vi "Controls - By List.vi"(7 "Msg Chain":string, 8 "error in (no error)":errorcluster {"code" format="Error %.0f"}, 10 "Controls Docs":refnum<class "GUI Documentation.lvclass">[](array[class]), 11 "VIDoc Printer - Confluence In":refnum<class "VIDoc Printer - Confluence.lvclass">) -> (0 "error out":errorcluster {"code" format="Error %.0f"}, 3 "VIDoc Printer - Confluence Out":refnum<class "VIDoc Printer - Confluence.lvclass">)   [LabVIEW 2023, in "VIDoc Printer - Confluence.lvlib" / "VIDoc Printer - Confluence.lvclass"]
uses:
  VIDoc Printer - Confluence.lvclass
  C:/projects/DMC/GitHub/DMC CLI VIDoc/Source/Documentation Generation/Printers/Printer/VIDoc Printer.lvclass
  Parsing/GUI Documentation/GUI Documentation.lvclass
  Confluence Formatting/Types/Format Combo Box.ctl
  Printer/VIDoc Printer.lvclass/VIDoc Printer.ctl
  VIDoc Printer - Confluence.lvclass/VIDoc Printer - Confluence.ctl
  Parsing/GUI Documentation/GUI Documentation.lvclass/GUI Documentation.ctl
  Types/VI Method Types.ctl
  Parsing/GUI Documentation/Get VI Info.vi
  Printer/Accessors/Get Formatting Settings - Bookmark Options.vi
  Printer/Accessors/Get Controls Settings - List Detail Level.vi
  Accessors/Get Sortable Tables.vi
  Accessors/Get Temporary Image Directory+.vi
  Accessors/Get Ctrls By List Expand.vi
  <vilib>/Utility/libraryn.llb/Create Directory Recursive.vi
  Confluence Formatting/Confluence Formatting.lvlib
  Printer/VIDoc Printer.lvclass
  UI Interaction/UI Interaction.lvclass
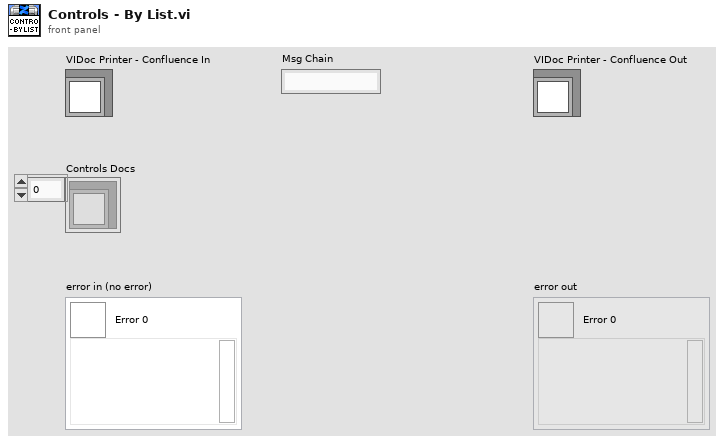
[diagram p1: front panel]
types:
  T1 = typedef "Confluence Formatting.lvlib/Format Combo Box.ctl" = string
  T2 = typedef "VIDoc Printer.lvlib/Printer Settings.lvclass/Bookmark Options.ctl" = cluster{"Bookmarks as New Line in VI Descriptions":bool, "Unique Bookmark Tags Only":bool, "Include Tag and Text":bool}
  T3 = typedef "VIDoc Printer.lvlib/Printer Settings.lvclass/Detail Level Enum.ctl" = enum16{"None", "Minimal", "Standard", "Full"}
  T4 = typedef "VIDoc Printer - Confluence.lvlib/VIDoc Printer - Confluence.lvclass/VI Method Types.ctl" = enum16{"Library", "Class", "Interface", "LLB", "UI", "List"}
  T5 = typedef "VIDoc Parsing.lvlib/Method Spec Cluster.ctl" = cluster{"VI Type Ext":T6, "Name":string, "Path":path, "Get Conpane Image":T7, "Description":string, "Get Library Access Scope":enum32{"invalid scope", "public", "private", "protected", "community"}, "Dispatch":T8, "ContainsCompiledCode":bool, "Exec.IsReentrant":bool, "Exec.ReentrancyType":enum16{"Share clones between instances", "Preallocate clone for each instance"}, "ExecInlining":bool, "ExecInlineIfPossible":bool, "Auto Err Handling":bool, "CodeComplexity":sgl, "Bookmark Tags":string[], "Control VI Type":enum32{"not a control VI", "control", "typedef", "strict typedef"}, "Controls":T9[], "VI Type":enum32{"invalid VI type", "Standard VI", "Control VI", "Global VI", "Polymorphic VI", "Configuration VI", "SubSystem", "Facade VI", "Method VI", "Statechart Diagram VI"}, "Minimum Size":T11, "Front Panel Window:Title":string, "Front Panel Window:Behavior":enum32{"Invalid", "Default", "Floating", "Floating/Auto-Hide", "Modal"}, "Front Panel Window:Closeable":bool, "Must Override":bool, "Must Use Parent Implementation":bool, "VI Icon":T7, "Front Panel":T7, "History:Revision Number":u32, "Metrics:Total Data Size":u32, "Execution:Allow Debugging":bool, "Execution:Preferred Exec System":enum32{"invalid execution system", "user interface", "standard", "instrument i/o", "data acquisition", "other 1", "other 2", "same as caller"}, "Execution:Priority":enum32{"invalid priority", "background priority", "normal priority", "above normal priority", "high priority", "time critical priority", "subroutine"}, "BM Tag Text":string[], "Block Diagram":T7, "Structure Tree":T12[]}
  T6 = typedef "VIDoc Parsing.lvlib/VI Type Extended Enum.ctl" = enum16{"Unknown", "Class Method", "Class Accessor Get", "Class Accessor Set", "Class Control", "Library Method", "Library Control", "VI", "Control"}
  T7 = typedef "imagedata.ctl" = cluster{"image type":i32, "image depth":i32, "image":u8[], "mask":u8[], "colors":u32[], "Rectangle":cluster{"left":i16, "top":i16, "right":i16, "bottom":i16}}
  T8 = typedef "VIDoc Parsing.lvlib/Class Dispatch Type Enum.ctl" = enum16{"None", "Static", "Dynamic"}
  T9 = typedef "VIDoc Parsing.lvlib/Controls Info Cluster.ctl" = cluster{"Name":string, "Description":string, "Data Type":string, "Tip Strip":string, "UID":i32, "Image Data":T7, "ToggleKeyBind":T10, "Raw Label":string, "Raw Caption":string}
  T10 = typedef "LVKeyTypeDef.ctl" = cluster{"Focus":bool, "Control":bool, "Shift":bool, "Key":string}
  T11 = typedef "LVPointTypeDef.ctl" = cluster{"Horizontal":i16, "Vertical":i16}
  T12 = typedef "VIDoc Parsing.lvlib/Structure Reporter.lvlib/Tree Cluster.ctl" = cluster{"Object Class Name":string, "Labels":string[], "Child Tag":string, "Item Indent":i32, "Child Only?":bool, "Glyph Index":i32}
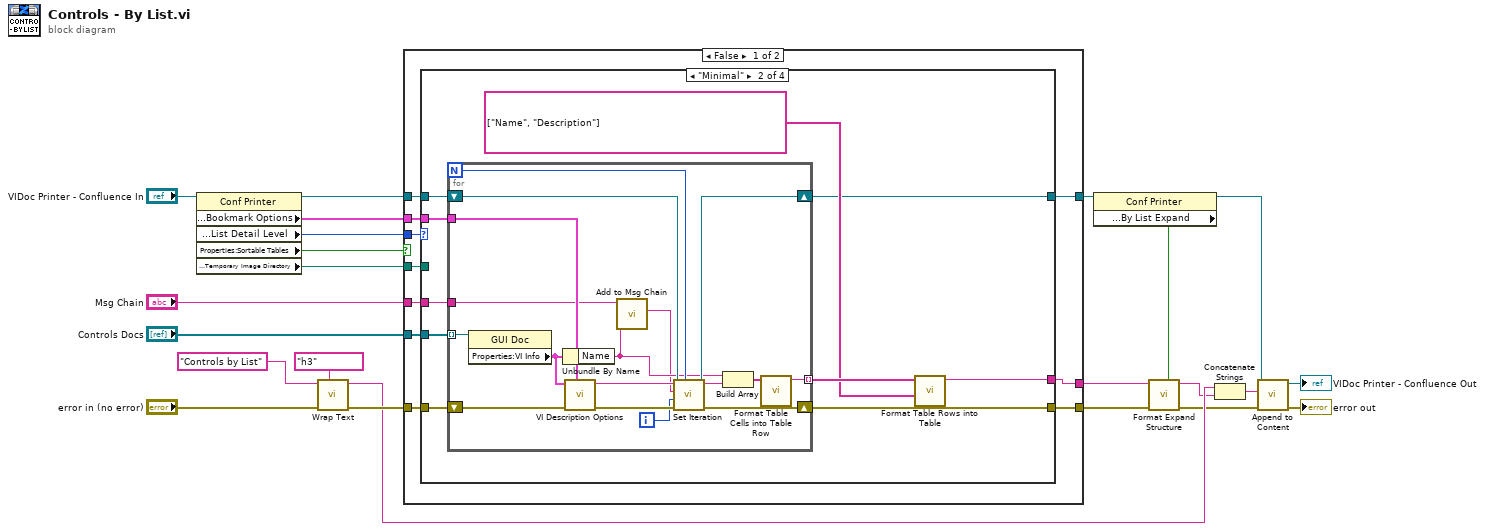
[diagram p0: block diagram]
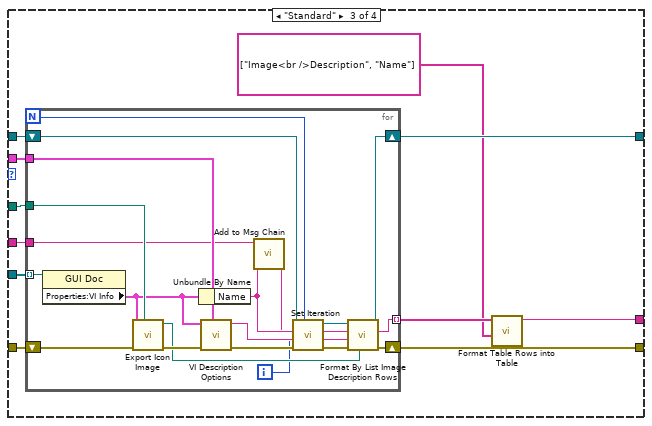
[diagram p3: hidden frame]
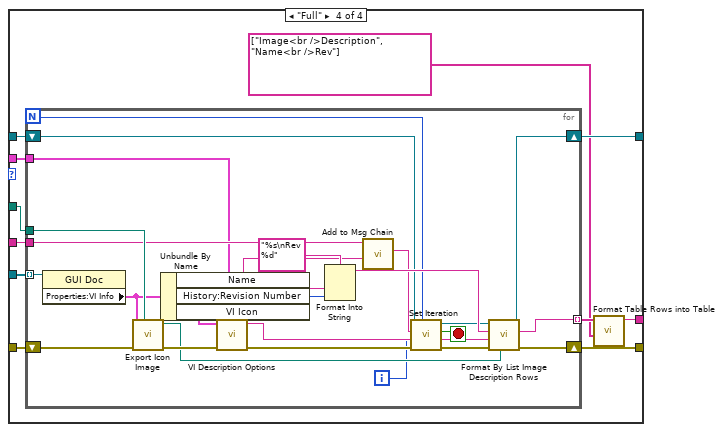
[diagram p4: hidden frame]
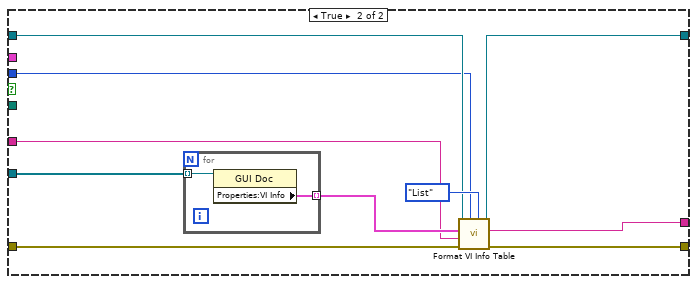
[diagram p5: hidden frame]
diagram:
  n1 = property class="Conf Printer"(reference="VIDoc Printer - Confluence In") -> (reference out=w20:refnum<class "VIDoc Printer - Confluence.lvclass">, "Properties:Settings:Formatting Options:Bookmark Options"=w9:T2, "Properties:Settings:Control Members:List Detail Level"=w8:T3, "Properties:Sortable Tables"=w2:bool, "Properties:Temporary Image Directory"=w1:path)  [unwired: 1 in, 1 out]
  n2 = call "Wrap Text.vi"("Formatting"=T1 "h3", "Error in"="error in (no error)", "String"="Controls by List" ("format string")) -> ("Error out"=w22:errorcluster, "Wrapped String"=w17:string)  [unwired: 7 in]
  n3 = case shown="False" w2 {
    tunnel: w22 -> [w33 w135]
    tunnel: [w32 w134] -> w21
    tunnel: w20 -> [w31 w132]
    tunnel: [w30 w128] -> w19
    tunnel: w1 -> [w29 _]
    tunnel: "Controls Docs" -> [w28 w129]
    tunnel: "Msg Chain" -> [w27 w130]
    tunnel: w9 -> [w26 _]
    tunnel: w8 -> [w25 w131]
    tunnel: [w24 w133] -> w6
    frame False {
      n4 = case shown="\"Minimal\"" w25 {
        tunnel: w33 -> [w35 w44 w71 w102]
        tunnel: [w35 w41 w65 w96] -> w32
        tunnel: w28 -> [_ w45 w72 w103]
        tunnel: [_ w42 w67 w98] -> w24
        tunnel: w31 -> [w34 w39 w69 w100]
        tunnel: [w34 w38 w68 w99] -> w30
        tunnel: w29 -> [_ _ w70 w101]
        tunnel: w27 -> [_ w37 w63 w94]
        tunnel: w26 -> [_ w36 w62 w93]
        frame "None", Default {
        }
        frame "Minimal" {
          n5 = for {
            N -> [w50]
            tunnel: w45 -> [w61] mode=indexing
            tunnel: w36 -> [w59]
            shift-right: [w53] -> w41
            shift-left: w44 -> [w58]
            tunnel: [w55] -> w43 mode=indexing
            shift-right: [w51] -> w38
            shift-left: w39 -> [w52]
            tunnel: w37 -> [w48]
            i -> [w49]
            n6 = property class="GUI Doc"(reference=w61) -> ("Properties:VI Info"=w60:T5)  [unwired: 1 in, 2 out]
            n7 = Unbundle By Name(w60) -> ("Name"=w47:string)
            n8 = call "VI Description Options.vi"("Bookmark Options"=w59, "Error in"=w58, "VI Info"=w60) -> ("Error out"=w54:errorcluster, "Description"=w57:string)  [unwired: 7 in]
            n9 = call "Add to Msg Chain.vi"("New"=w47, "Msg Chain in"=w48) -> ("Msg Chain out"=w46:string)  [unwired: 9 in]
            n10 = call "Set Iteration.vi"("Progress Max"=w50, "error in (no error)"=w54, "Progress Value"=w49, "Message (No Message Update)"=w46, "VIDoc Printer In"=w52) -> ("error out"=w53:errorcluster, "VIDoc Printer Out"=w51:refnum<class "VIDoc Printer - Confluence.lvclass">)  [unwired: 4 in, 1 out]
            n11 = Build Array(w47, w57) -> (w56:string[])
            n12 = call "Format Table Cells into Table Row.vi"("Table Cells"=w56) -> ("Table Row Text"=w55:string)  [unwired: 10 in]
          }
          n13 = call "Format Table Rows into Table.vi"("Table Headers"=string[] ["Name", "Description"], "Table Rows"=w43) -> ("Table Text"=w42:string)  [unwired: 9 in]
        }
        frame "Standard" {
          n14 = for {
            N -> [w77]
            tunnel: w72 -> [w92] mode=indexing
            tunnel: w62 -> [w91]
            shift-right: [w86] -> w65
            shift-left: w71 -> [w89]
            tunnel: w70 -> [w90]
            shift-right: [w85] -> w68
            shift-left: w69 -> [w79]
            tunnel: [w82] -> w66 mode=indexing
            tunnel: w63 -> [w75]
            i -> [w76]
            n15 = property class="GUI Doc"(reference=w92) -> ("Properties:VI Info"=w87:T5)  [unwired: 1 in, 2 out]
            n16 = call "Export Icon Image.vi"("Temporary Image Directory"=w90, "Error in"=w89, "VI Info"=w87) -> ("Error out"=w88:errorcluster, "Image Path"=w83:path)  [unwired: 7 in]
            n17 = Unbundle By Name(w87) -> ("Name"=w74:string)
            n18 = call "VI Description Options.vi"("Bookmark Options"=w91, "Error in"=w88, "VI Info"=w87) -> ("Error out"=w81:errorcluster, "Description"=w84:string)  [unwired: 7 in]
            n19 = call "Add to Msg Chain.vi"("New"=w74, "Msg Chain in"=w75) -> ("Msg Chain out"=w73:string)  [unwired: 9 in]
            n20 = call "Set Iteration.vi"("Progress Max"=w77, "error in (no error)"=w81, "Progress Value"=w76, "Message (No Message Update)"=w73, "VIDoc Printer In"=w79) -> ("error out"=w80:errorcluster, "VIDoc Printer Out"=w78:refnum<class "VIDoc Printer - Confluence.lvclass">)  [unwired: 4 in, 1 out]
            n21 = call "Format By List Image Description Rows.vi"("Image"=w83, "error in (no error)"=w80, "Description"=w84, "Name"=w74, "VIDoc Printer - Confluence In"=w78) -> ("error out"=w86:errorcluster, "Table Rows Text"=w82:string, "VIDoc Printer - Confluence Out"=w85:refnum<class "VIDoc Printer - Confluence.lvclass">)  [unwired: 3 in, 1 out]
          }
          n22 = call "Format Table Rows into Table.vi"("Table Headers"=string[] ["Image<br />Description", "Name"], "Table Rows"=w66) -> ("Table Text"=w67:string)  [unwired: 9 in]
        }
        frame "Full" {
          n23 = for {
            N -> [w110]
            tunnel: w103 -> [w127] mode=indexing
            shift-right: [w122] -> w96
            shift-left: w102 -> [w125]
            tunnel: w101 -> [w126]
            shift-right: [w121] -> w99
            shift-left: w100 -> [w112]
            tunnel: [w118] -> w97 mode=indexing
            tunnel: w94 -> [w108]
            tunnel: w93 -> [w104]
            i -> [w109]
            stop <- w105 stop-if-true
            n24 = property class="GUI Doc"(reference=w127) -> ("Properties:VI Info"=w123:T5)  [unwired: 1 in, 2 out]
            n25 = call "Export Icon Image.vi"("Temporary Image Directory"=w126, "Error in"=w125, "VI Info"=w123) -> ("Error out"=w124:errorcluster, "Image Path"=w119:path)  [unwired: 7 in]
            n26 = Unbundle By Name(w123) -> ("Name"=w107:string, "History:Revision Number"=w116:u32)  [unwired: 1 out]
            n27 = call "VI Description Options.vi"("Bookmark Options"=w104, "Error in"=w124, "VI Info"=w123) -> ("Error out"=w114:errorcluster, "Description"=w120:string)  [unwired: 7 in]
            n28 = Format Into String(format string="%s\nRev %d", w107, w116) -> (resulting string=w115:string)  [unwired: 2 in, 1 out]
            n29 = call "Add to Msg Chain.vi"("New"=w107, "Msg Chain in"=w108) -> ("Msg Chain out"=w106:string)  [unwired: 9 in]
            n30 = call "Set Iteration.vi"("Progress Max"=w110, "error in (no error)"=w114, "Progress Value"=w109, "Message (No Message Update)"=w106, "VIDoc Printer In"=w112) -> ("error out"=w113:errorcluster, "Abort?"=w105:bool, "VIDoc Printer Out"=w111:refnum<class "VIDoc Printer - Confluence.lvclass">)  [unwired: 4 in]
            n31 = call "Format By List Image Description Rows.vi"("Image"=w119, "error in (no error)"=w113, "Description"=w120, "Name"=w115, "VIDoc Printer - Confluence In"=w111) -> ("error out"=w122:errorcluster, "Table Rows Text"=w118:string, "VIDoc Printer - Confluence Out"=w121:refnum<class "VIDoc Printer - Confluence.lvclass">)  [unwired: 3 in, 1 out]
          }
          n32 = call "Format Table Rows into Table.vi"("Table Headers"=string[] ["Image<br />Description", "Name<br />Rev"], "Table Rows"=w97) -> ("Table Text"=w98:string)  [unwired: 9 in]
        }
      }
    }
    frame True {
      n33 = for {
        tunnel: w129 -> [w139] mode=indexing
        tunnel: [w138] -> w136 mode=indexing
        n34 = property class="GUI Doc"(reference=w139) -> ("Properties:VI Info"=w138:T5)  [unwired: 1 in, 2 out]
      }
      n35 = call "Format VI Info Table.vi"("Type"=VI_Method_Types."List", "Methods"=w131, "Error in"=w135, "Msg Chain"=w130, "VI Info Array"=w136, "VIDoc Printer - Confluence In"=w132) -> ("Error out"=w134:errorcluster, "Table String"=w133:string, "VIDoc Printer - Confluence Out"=w128:refnum<class "VIDoc Printer - Confluence.lvclass">)  [unwired: 3 in]
    }
  }
  n36 = property class="Conf Printer"(reference=w19) -> (reference out=w4:refnum<class "VIDoc Printer - Confluence.lvclass">, "Properties:Expand?:Control:By List Expand"=w3:bool)  [unwired: 1 in, 1 out]
  n37 = call "Format Expand Structure.vi"("Enable? (T)"=w3, "Error in"=w21, "Content"=w6) -> ("Error out"=w7:errorcluster, "Expand String"=w5:string)  [unwired: 7 in]
  n38 = Concatenate Strings(w17, w5) -> (w18:string)
  n39 = call "Append to Content.vi"("error in (no error)"=w7, "Content"=w18, "VIDoc Printer - Confluence In"=w4) -> ("error out"=→"error out":errorcluster, "VIDoc Printer - Confluence Out"=→"VIDoc Printer - Confluence Out":refnum<class "VIDoc Printer - Confluence.lvclass">)  [unwired: 7 in]
